vi "About.vi"() -> ()   [LabVIEW 2010]
doc: "This VI is used to illustrate the About box capability with LabVIEW executables."
panel:
  out "error out":errorcluster
  in  "error in (no error)":errorcluster
  # "LabVIEW\n\n\n\n\n\n\nCopyright ©2010 National Instruments Corporation.  All Rights Reserved."
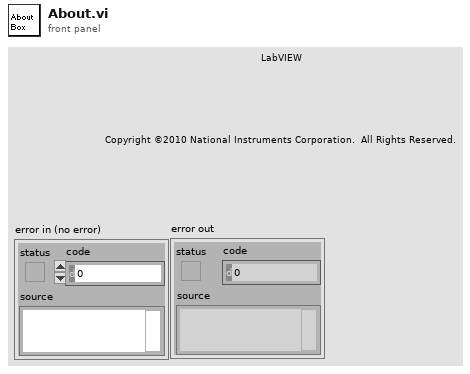
[diagram p1: front panel]
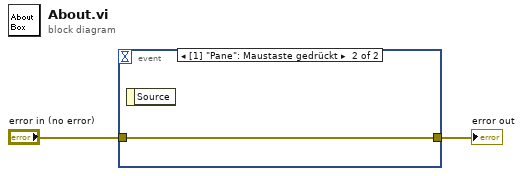
[diagram p0: block diagram]
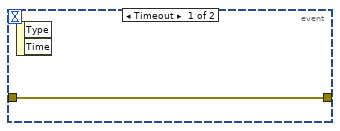
[diagram p2: hidden frame]
diagram:
  n1 = event shown="[1] \"Pane\": Maustaste gedrückt" {
    selector: _ -> [_ _]
    dyn-events: _ -> [_ _]
    timeout: _ -> [_ _]
    tunnel: [w3 w4] -> w2
    tunnel: "error in (no error)" -> [w3 w4]
    event Timeout {
      n2 = event-data() -> ()  [unwired: 1 in, 2 out]
    }
    event Mouse Down {
      n3 = event-data() -> ()  [unwired: 1 in, 1 out]
    }
  }
  "error out" <- w2
